vi "CumplimientoFrecuencia.vi"(8 "error in (no error)":errorcluster, 11 "Prueba21_1 in":refnum<class "Prueba21.lvclass">) -> (0 "error out":errorcluster, 3 "Prueba21_1 out":refnum<class "Prueba21.lvclass">)   [LabVIEW 2019, in "Prueba21.lvclass"]
uses:
  Prueba21.lvclass
  Prueba21.lvclass/Prueba21.ctl
panel:
  out "cumpimiento":string
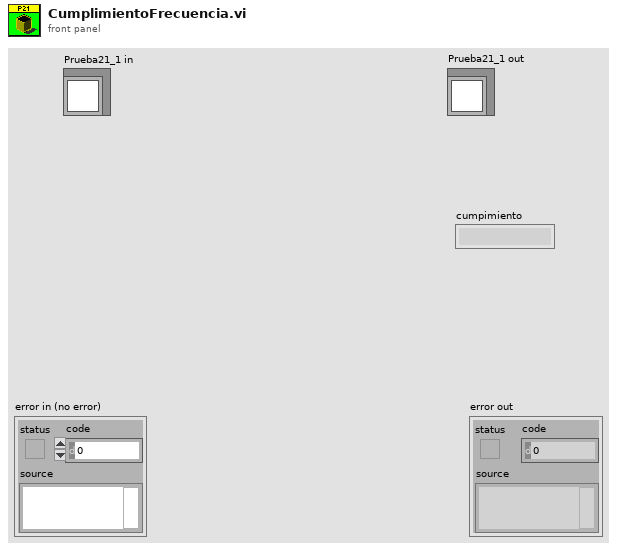
[diagram p1: front panel]
types:
  T1 = cluster{"ControlName":string, "ControlReference":refnum<vi>}[]
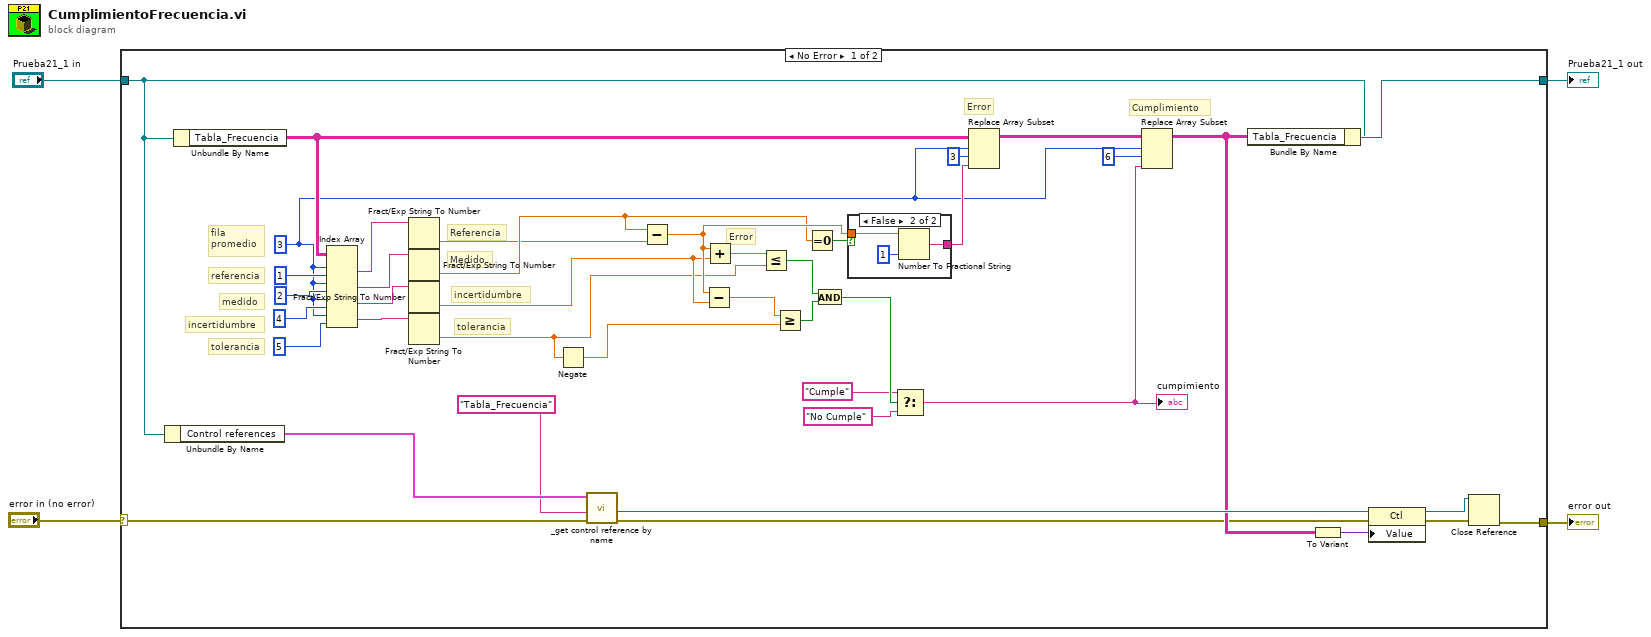
[diagram p0: block diagram]
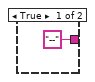
[diagram p2: hidden frame]
diagram:
  n1 = case shown="No Error" "error in (no error)" {
    selector: "error in (no error)" -> [w5 w51]
    tunnel: [w7 w51] -> w3
    tunnel: [w31 w50] -> w2
    tunnel: "Prueba21_1 in" -> [w15 w50]
    frame No Error {
      w21 = 3 ("index (row)")
      # "tolerancia"
      # "incertidumbre"
      # "Medido"
      # "Referencia"
      # "tolerancia"
      # "incertidumbre"
      # "medido"
      # "referencia"
      # "fila\npromedio"
      # "Cumplimiento"
      # "Error"
      # "Error"
      n2 = Unbundle By Name(w15) -> ("Control references"=w14:T1)
      n3 = Unbundle By Name(w15) -> ("Tabla_Frecuencia"=w29:string[][])
      n4 = Index Array(array=w29, index (row) #1=w21, index (col) #1=1 ("disabled index (col)"), index (row) #2=w21, index (col) #2=2 ("disabled index (col)"), index (row) #3=w21, index (col) #3=4 ("disabled index (col)"), index (row) #4=w21, index (col) #4=5 ("disabled index (col)")) -> (element #1=w25:string, element #2=w24:string, element #3=w23:string, element #4=w22:string)
      n5 = Fract/Exp String To Number(string=w25) -> (number=w19:dbl)  [unwired: 3 in, 1 out]
      n6 = Fract/Exp String To Number(string=w24) -> (number=w20:dbl)  [unwired: 3 in, 1 out]
      n7 = Fract/Exp String To Number(string=w23) -> (number=w18:dbl)  [unwired: 3 in, 1 out]
      n8 = Fract/Exp String To Number(string=w22) -> (number=w16:dbl)  [unwired: 3 in, 1 out]
      n9 = Negate(x=w16) -> (-x=w17:dbl)
      n10 = call "_get control reference by name.vi"("error in (no error)"=w5, "Control name"="Tabla_Frecuencia", "Control references"=w14) -> ("error out"=w6:errorcluster, "Ctl Refnum"=w12:refnum<vi>)  [unwired: 3 in]
      n11 = Subtract(x=w20, y=w19) -> (x-y=w32:dbl)
      n12 = Subtract(x=w32, y=w18) -> (x-y=w42:dbl)
      n13 = Add(x=w32, y=w18) -> (x+y=w45:dbl)
      n14 = Less Or Equal?(x=w45, y=w16) -> (x <= y?=w44:bool)
      n15 = Greater Or Equal?(x=w42, y=w17) -> (x >= y?=w43:bool)
      n16 = Equal To 0?(x=w20) -> (x = 0?=w33:bool)
      n17 = And(x=w44, y=w43) -> (x .and. y?=w41:bool)
      n18 = case shown="False" w33 {
        tunnel: w32 -> [_ w49]
        tunnel: ["--" w47] -> w34
        frame True {
        }
        frame False {
          n19 = Number To Fractional String(number=w49, precision (6)=i16 1) -> (F-format string=w47:string)  [unwired: 2 in]
        }
      }
      n20 = Select(t="Cumple", s=w41, f="No Cumple") -> (s? t:f=w38:string)
      "cumpimiento" <- w38
      n21 = Replace Array Subset(array=w29, new element=w34, index (row)=w21, index (col)=3 ("disabled index (col)")) -> (w36:string[][])
      n22 = Replace Array Subset(array=w36, new element=w38, index (row)=w21, index (col)=6 ("index (row)")) -> (w10:string[][])
      n23 = Bundle By Name(cluster=w15, "Tabla_Frecuencia"=w10) -> (w31:refnum<class "Prueba21.lvclass">)
      n24 = To Variant(anything=w10) -> (Variant=w11:variant)
      n25 = property on="Property Node" class="Ctl"(reference=w12, error in=w6, "Value"=w11) -> (reference out=w9:refnum<vi>, error out=w8:errorcluster)
      n26 = Close Reference(reference=w9, error in (no error)=w8) -> (error out=w7:errorcluster)
    }
    frame Error {
    }
  }
  "error out" <- w3
  "Prueba21_1 out" <- w2
